vi "Get Config.vi"(8 "error in (no error)":errorcluster, 11 "DriverMasterAsync in":refnum<class "DriverMasterAsync.lvclass">) -> (0 "error out":errorcluster, 1 "Config Data":variant, 3 "DriverMasterAsync out":refnum<class "DriverMasterAsync.lvclass">)   [LabVIEW 2014, in "DriverMasterAsync.lvlib" / "DriverMasterAsync.lvclass"]
uses:
  DriverMasterAsync.lvclass
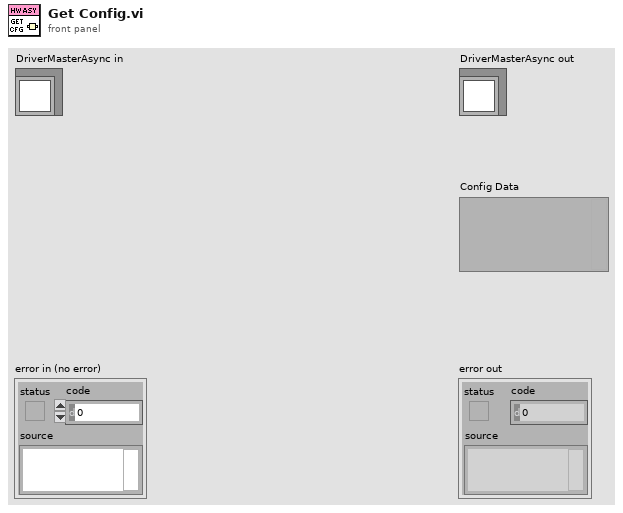
[diagram p1: front panel]
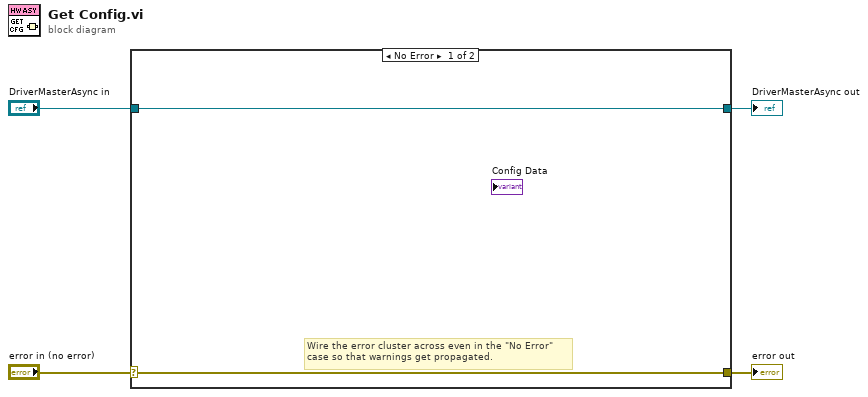
[diagram p0: block diagram]
diagram:
  n1 = case shown="No Error" "error in (no error)" {
    selector: "error in (no error)" -> [w5 w8]
    tunnel: [w5 w8] -> w3
    tunnel: [w6 w7] -> w1
    tunnel: "DriverMasterAsync in" -> [w6 w7]
    frame No Error {
      # "Wire the error cluster across even in the \"No Error\"\ncase so that warnings get propagated."
    }
    frame Error {
    }
  }
  "error out" <- w3
  "DriverMasterAsync out" <- w1
